vi "Springboard MAIN - App.vi"() -> ()   [LabVIEW 2022 SP3, in "Springboard TLB`.lvlib" / "Springboard TLB`.lvclass"]
uses:
  Springboard TLB`.lvclass
  Application Components/Trigger API/System Trigger.ctl
  State Machine/State.ctl
  Core Components/Error Handler/TLB` Error Handler.lvclass
  Application Components/Configuration/Springboard Station Configuration.lvclass
  Springboard TLB`.lvclass/Springboard TLB`.ctl
  <vilib>/Utility/sysdir.llb/System Directory Type.ctl
  <vilib>/Utility/error.llb/Trim Whitespace One-Sided.vi
  <vilib>/Utility/error.llb/Error Cluster From Error Code.vi
  <vilib>/ErrorRing/Error Ring.xnode
  <vilib>/regexp/Match Regular Expression.xnode
  Application Components/Trigger API/Springboard Trigger API.lvlib
  Springboard TLB`.lvlib
  Core Components/Actions/Actions.lvlib
  Core Components/Dependencies/TLB`_Dependencies.lvlib
  <vilib>/Utility/config.llb/NI_LVConfig.lvlib
panel:
  out "Application Name":string
  out "Application:All Libraries in Application Instance":string[](array[string])
  in  "Library Path":path=path "C:/Program Files (x86)/National Instruments/LabVIEW 2018/project/TLB`/_Dependencies/TLB` Template"
  in  "Add to Project":u16(ring)=2 items=["TLB` Springboard.lvproj", "Untitled Project 14", "< Create In New Project... >"]
  in  "Cancel":bool
  in  "Build":bool
  in  "New TLB Name":string
  in  "Destination Folder":path=path "C:/Users/Public/Documents"
  out "error out":errorcluster
  out "State":string
  out "Status":string
  # "Description"
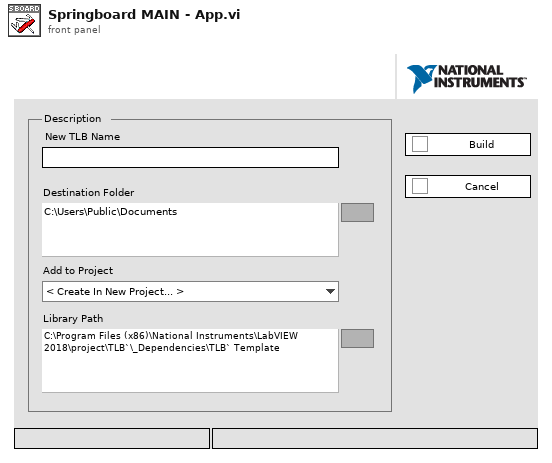
[diagram p1: front panel]
types:
  T1 = typedef "Springboard TLB`.lvlib/Springboard TLB`.lvclass/State.ctl" = enum16{"<Startup>", "Idle", "Evaluate Build Directory", "Creating", "Evaluate Build", "<Shutdown>", "<Error>"}
  T2 = enum16{"Close Display", "Clear References", "Close Error Handler"}
  T3 = enum16{"Clear SR", "Set Display", "Set Shifter", "Initialize Events", "Init Q"}
  T4 = typedef "Springboard TLB`.lvlib/Springboard Trigger API.lvlib/System Trigger.ctl" = enum16{"<None>", "<Return to Safe State Actions>", "<Cache User Parameters>", "<Close Application>", "<Error>", "Create New", "Abort Creation", "Cancel"}
  T5 = typedef "Springboard TLB`.lvlib/_UI CORE Event References.ctl" = cluster{"Exit Event":refnum<user-event>, "State Indicator":refnum<user-event>, "Status Indicator":refnum<user-event>}
  T6 = typedef "Springboard TLB`.lvlib/_UI APP Event References.ctl" = cluster{"Exit Event":refnum<user-event>, "Application Name":refnum<user-event>}
  T7 = enum8{"Enabled", "Disabled", "Disabled and Grayed Out"}
  T8 = typedef "System Directory Type.ctl" = i32
  T9 = typedef "NI_LVConfig.lvlib/Config Data RefNum.ctl" = refnum<k1>
  T10 = enum32{"Invalid", "Standard", "Closed", "Hidden", "Minimized", "Maximized"}
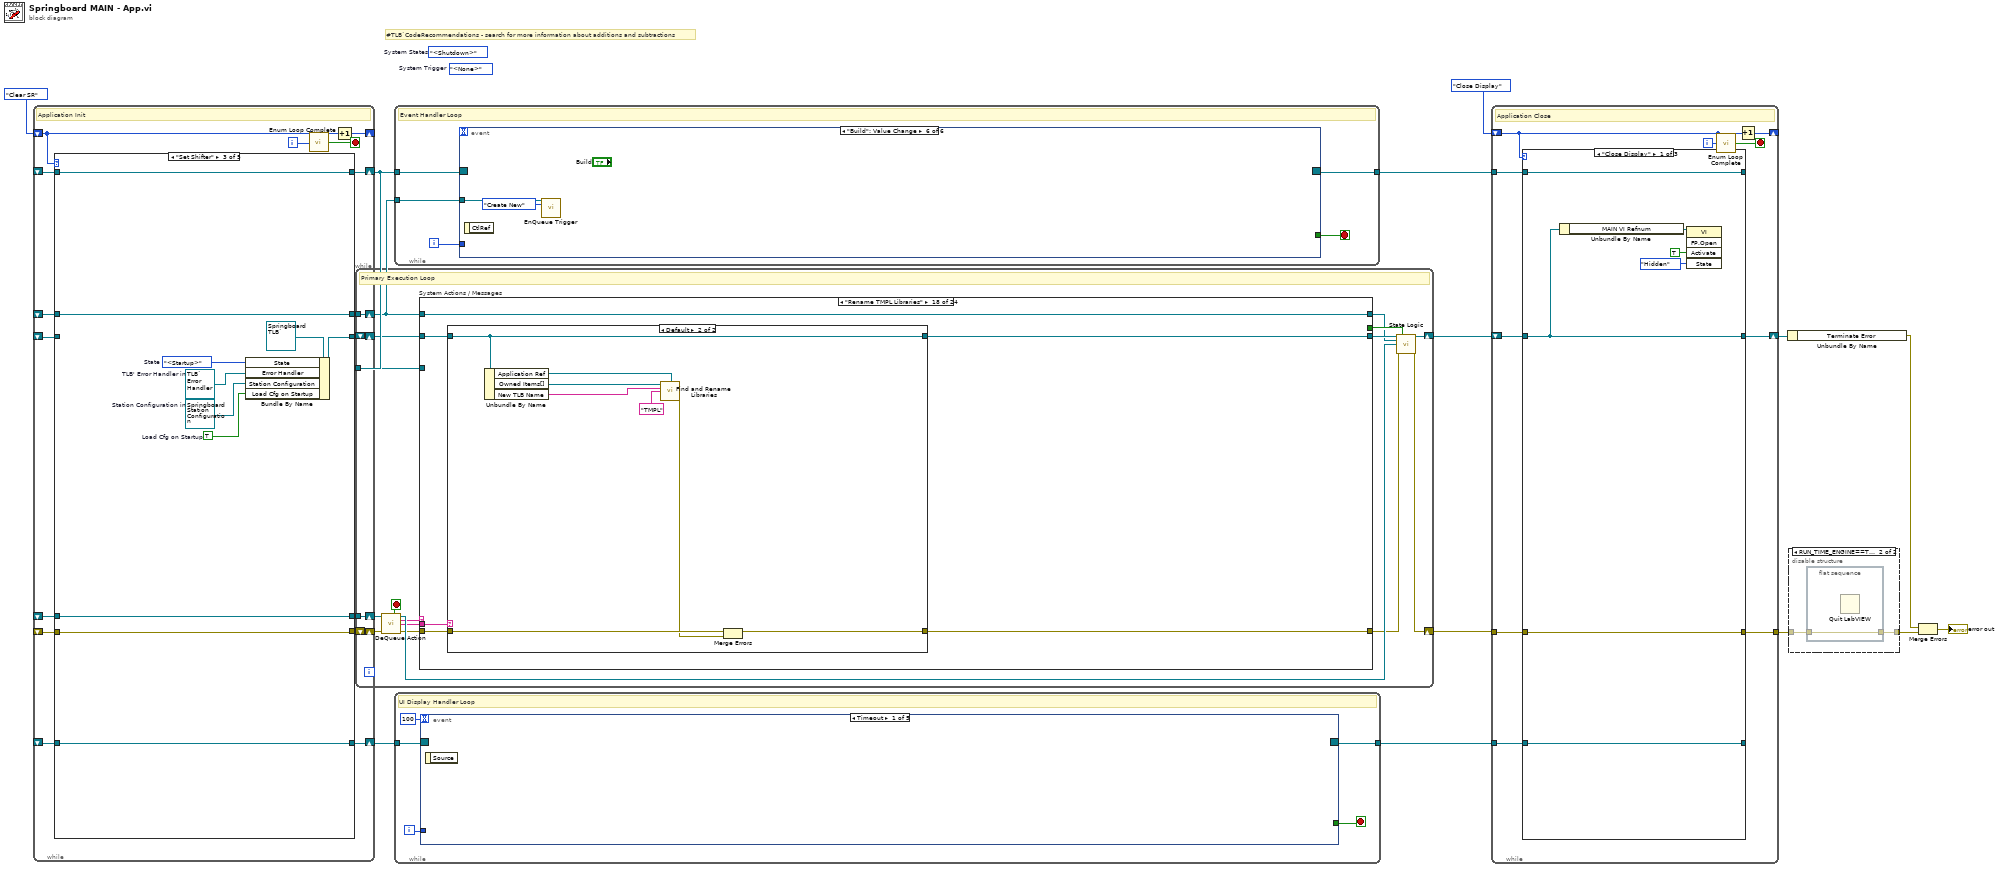
[diagram p0: block diagram]
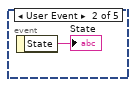
[diagram p2: hidden frame]
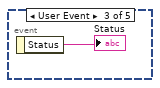
[diagram p3: hidden frame]
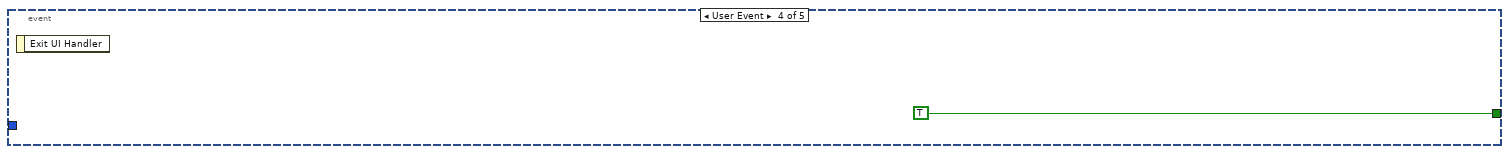
[diagram p4: hidden frame]
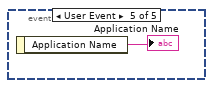
[diagram p5: hidden frame]
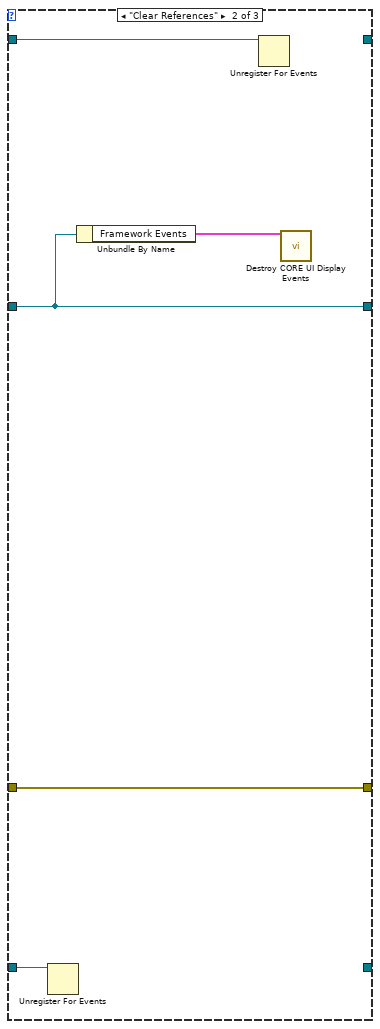
[diagram p7: hidden frame]
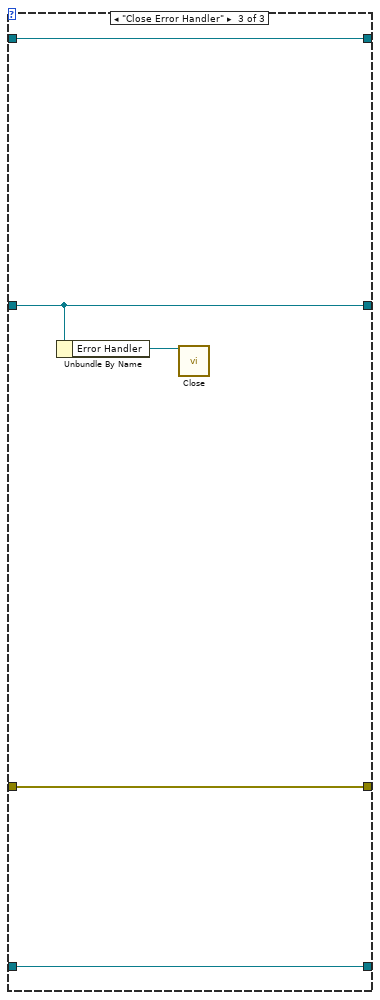
[diagram p8: hidden frame]
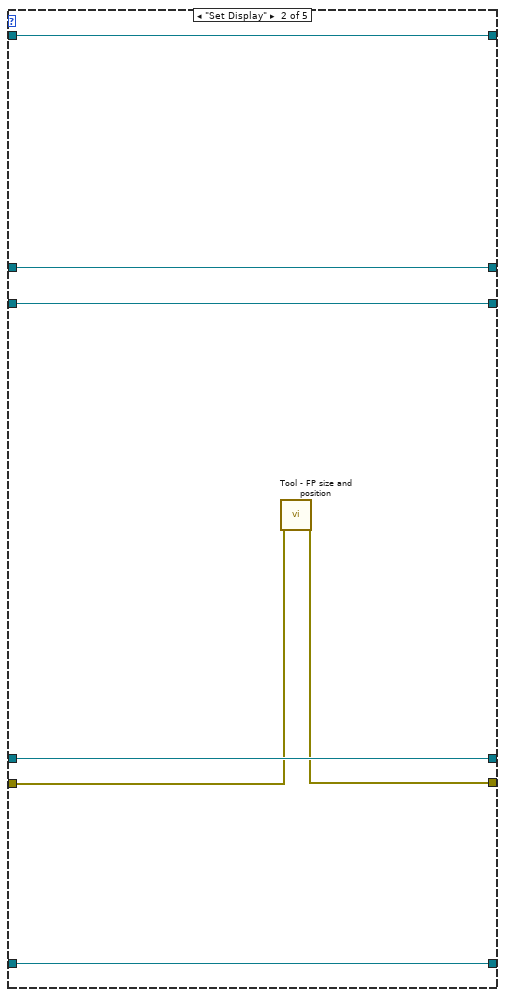
[diagram p10: hidden frame]
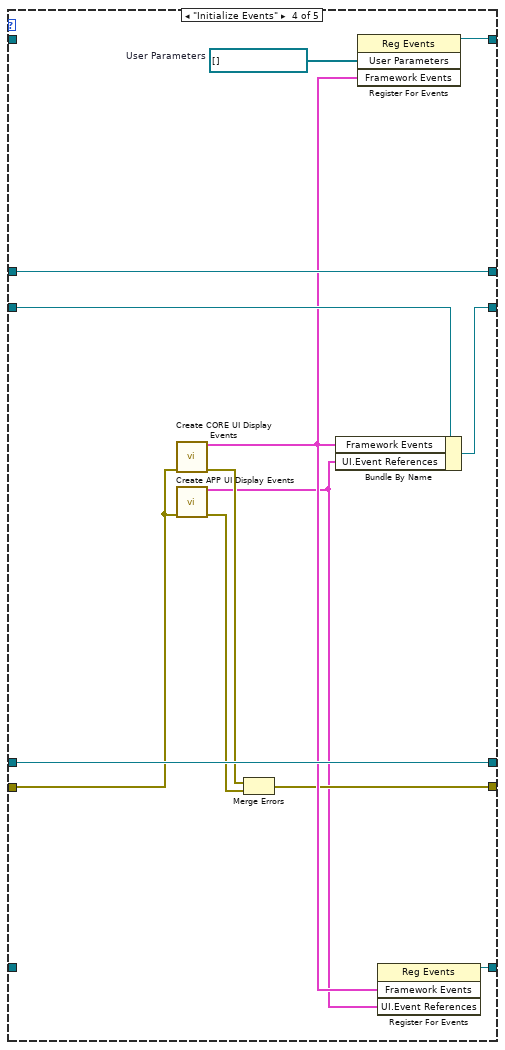
[diagram p11: hidden frame]
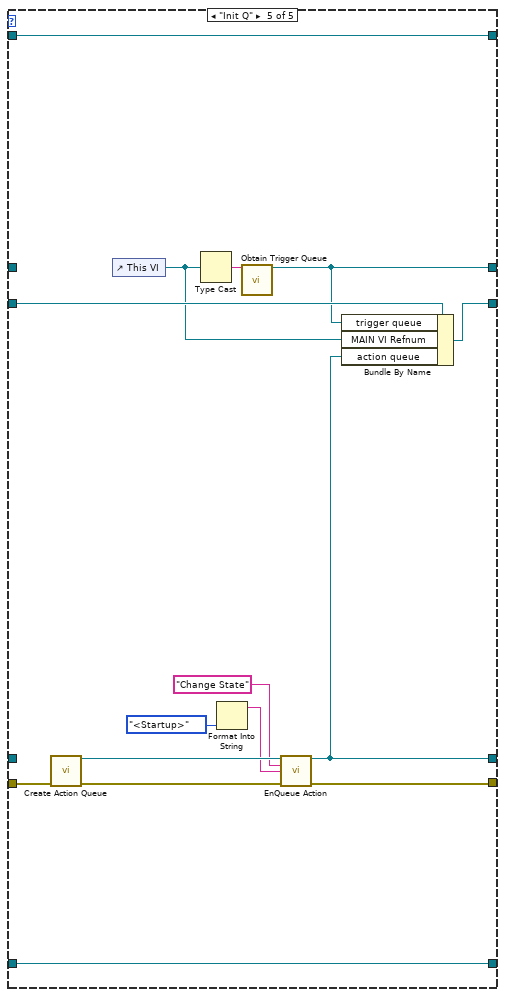
[diagram p12: hidden frame]
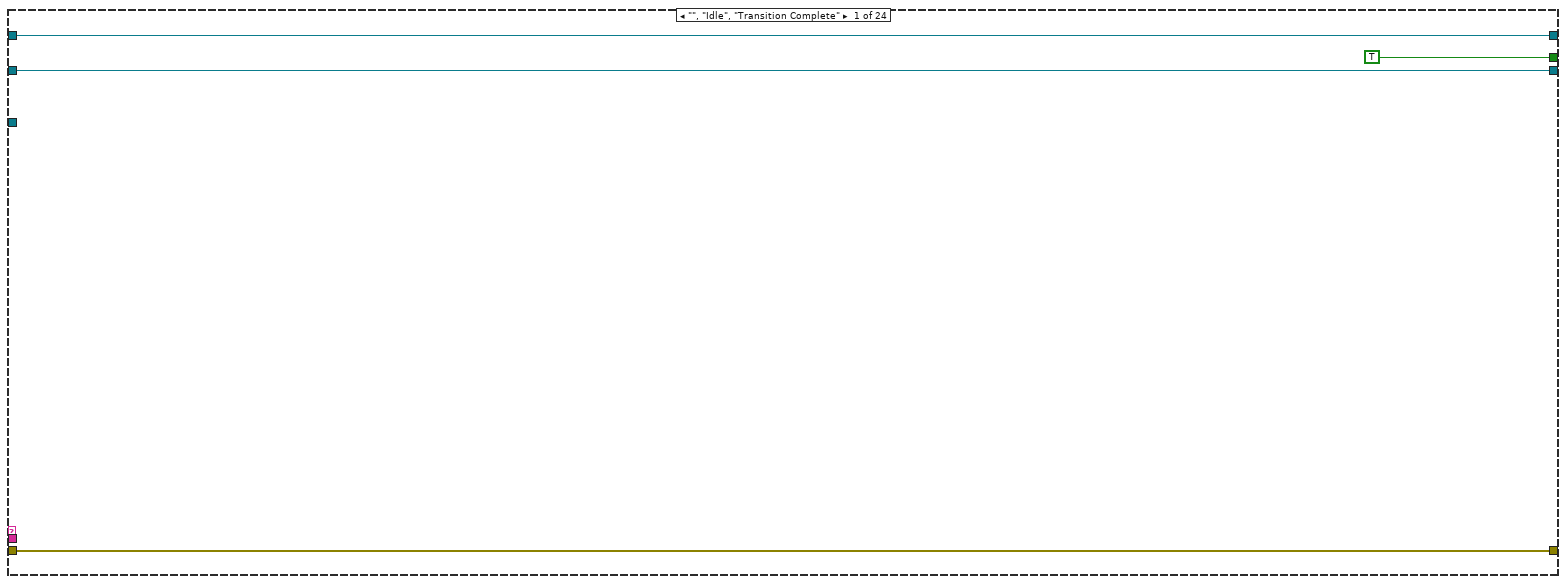
[diagram p13: hidden frame]
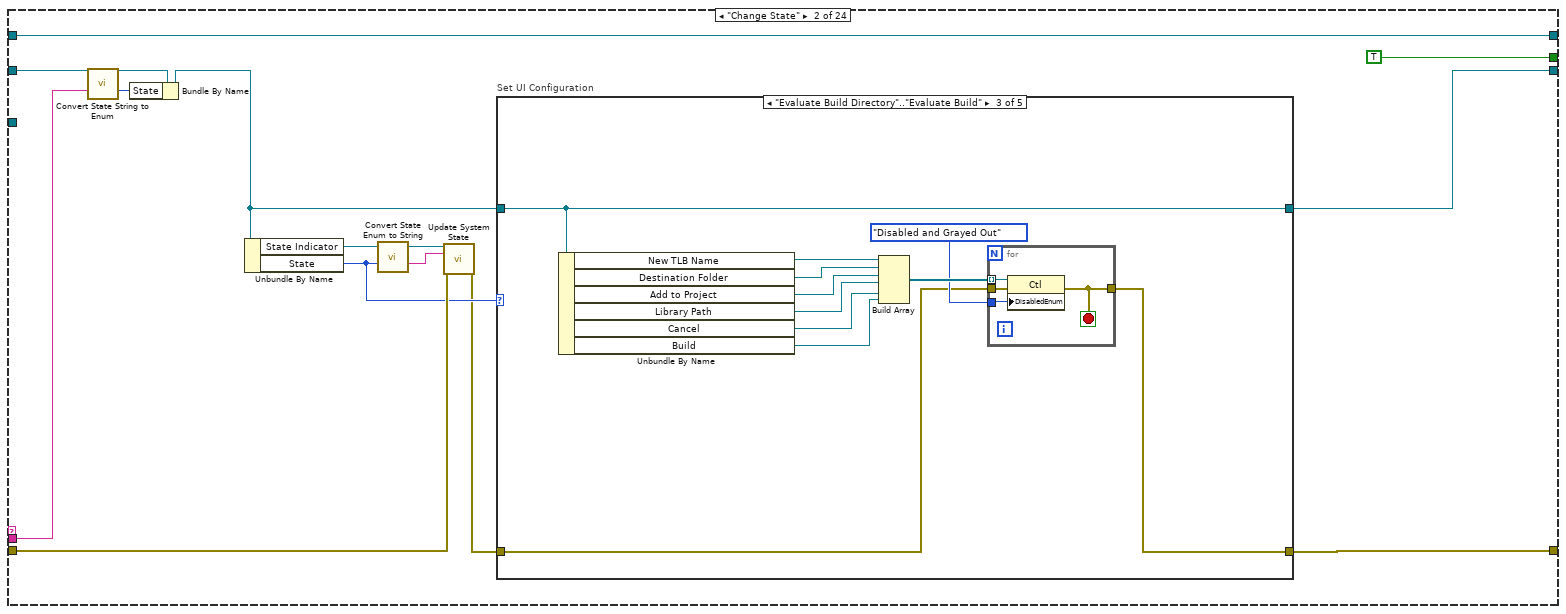
[diagram p14: hidden frame]
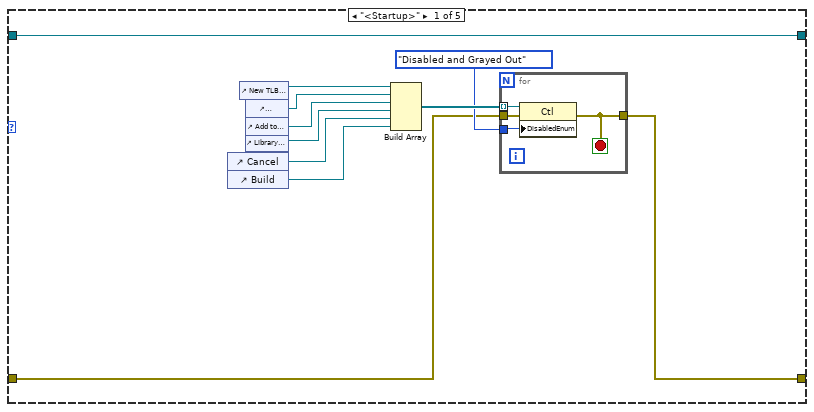
[diagram p15: hidden frame]
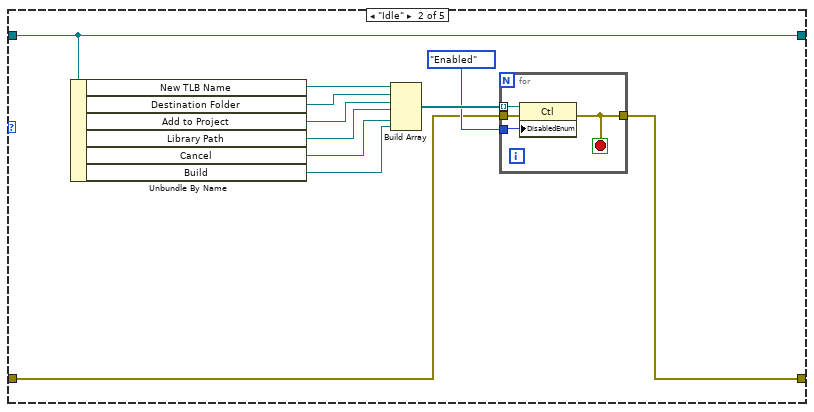
[diagram p16: hidden frame]
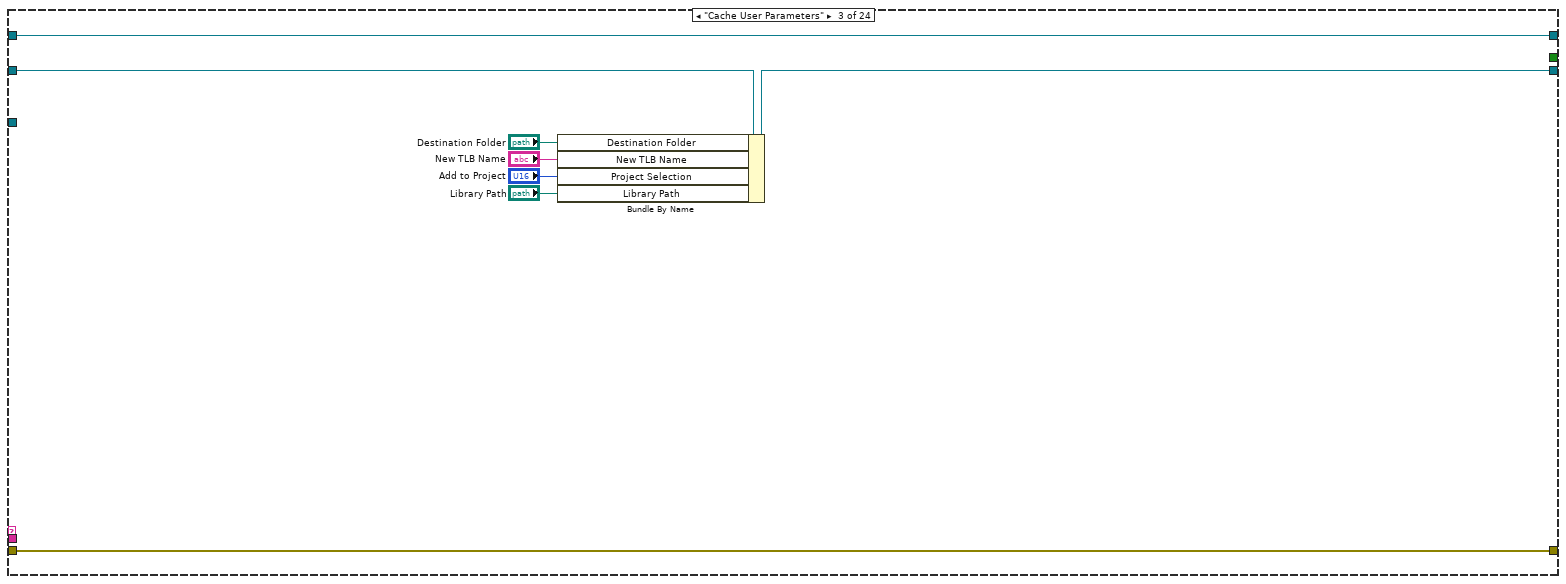
[diagram p19: hidden frame]
diagram:
  (unwired) State."<Shutdown>"  # System States
  (unwired) System_Trigger."<None>"  # System Trigger
  # "#TLB`CodeRecommendations - search for more information about additions and subtractions"
  n1 = while {
    shift-right: [w29] -> _
    shift-left: T3."Clear SR" -> [w18]
    shift-right: [w33] -> w17
    shift-left: _ -> [w28]
    shift-right: [w30] -> w12
    shift-left: _ -> [w27]
    shift-right: [w32] -> w11
    shift-left: _ -> [w26]
    shift-right: [w31] -> w10
    shift-left: _ -> [w25]
    shift-right: [w24] -> w6
    shift-left: _ -> [w23]
    shift-right: [w22] -> w9
    shift-left: _ -> [w21]
    i -> [w19]
    stop <- w20 stop-if-true
    # "Application Init"
    n2 = case shown="\"Set Shifter\"" w18 {
      tunnel: [_ w38 w51 w64 w68] -> w33
      tunnel: [_ w36 w50 w54 w72] -> w30
      tunnel: [_ w40 w46 w62 w77] -> w31
      tunnel: [_ w39 w49 w61 w79] -> w32
      tunnel: w28 -> [_ w38 w51 w64 _]
      tunnel: w27 -> [_ w37 w50 w53 w74]
      tunnel: w26 -> [_ w39 w49 _ w79]
      tunnel: w25 -> [_ w40 _ w63 w78]
      tunnel: [_ w35 w48 w60 w69] -> w24
      tunnel: w23 -> [_ w35 w48 w60 _]
      tunnel: [_ w34 w44 w58 w75] -> w22
      tunnel: w21 -> [_ w34 w44 _ w75]
      frame "Clear SR" {
      }
      frame "Set Display" {
        n3 = call "Tool - FP size and position.vi"("error in (no error)"=w37) -> ("error out"=w36:errorcluster)  [unwired: 17 in, 1 out]
      }
      frame "Set Shifter" {
        w41 = TRUE  # Load Cfg on Startup
        w42 = refnum<class "Springboard Station Configuration.lvclass"> refnum  # Station Configuration in
        w43 = refnum<class "TLB` Error Handler.lvclass"> refnum  # TLB' Error Handler in
        w47 = State."<Startup>"  # State
        n4 = Bundle By Name(cluster=refnum<class "Springboard TLB`.lvclass"> refnum ("TLB` Template.lvlib:TLB' Template.lvclass"), "State"=w47, "Error Handler"=w43, "Station Configuration"=w42, "Load Cfg on Startup"=w41) -> (w46:refnum<class "Springboard TLB`.lvclass">)
      }
      frame "Initialize Events" {
        w59 = refnum<vi>[] []  # User Parameters
        n5 = call "Create CORE UI Display Events.vi"("error in"=w53) -> ("Framework Events"=w57:T5, "error out"=w56:errorcluster)  [unwired: 13 in]
        n6 = call "Create APP UI Display Events.vi"("error in"=w53) -> ("UI.Event References"=w52:T6, "error out"=w55:errorcluster)  [unwired: 13 in]
        n7 = Merge Errors(w56, w55) -> (w54:errorcluster)
        n8 = Bundle By Name(cluster=w63, "Framework Events"=w57, "UI.Event References"=w52) -> (w62:refnum<class "Springboard TLB`.lvclass">)
        n9 = register-events(w59, w57) -> (reference out=w61:refnum<event-registration>)  [unwired: 2 in, 1 out]
        n10 = register-events(w57, w52) -> (reference out=w58:refnum<event-registration>)  [unwired: 2 in, 1 out]
      }
      frame "Init Q" {
        n11 = call "Create Action Queue.vi"("error in"=w74) -> ("action queue out"=w71:refnum<queue>, "error out"=w73:errorcluster)  [unwired: 13 in]
        n12 = control-ref of="This VI"() -> (w76:refnum<vi>)
        n13 = Type Cast(x=w76) -> (*(type *) &x=w70:string)  [unwired: 1 in]
        n14 = Format Into String(State."<Startup>" ("State")) -> (resulting string=w65:string)  [unwired: 3 in, 1 out]
        n15 = call "Obtain Trigger Queue.vi"("trigger queue name"=w70) -> ("trigger queue out"=w69:refnum<queue>)  [unwired: 13 in, 1 out]
        n16 = call "EnQueue Action.vi"("action queue in"=w71, "action"="Change State" ("Message Name"), "data in"=w65, "error in"=w73) -> ("action queue out"=w68:refnum<queue>, "error out"=w72:errorcluster)  [unwired: 10 in]
        n17 = Bundle By Name(cluster=w78, "trigger queue"=w69, "MAIN VI Refnum"=w76, "action queue"=w68) -> (w77:refnum<class "Springboard TLB`.lvclass">)
      }
    }
    n18 = call "Enum Loop Complete.vi"("Current State Enum"=w18, "Itteration"=w19) -> ("Loop Complete?"=w20:bool)  [unwired: 12 in, 1 out]
    n19 = Increment(x=w18) -> (x+1=w29:T3)
  }
  n20 = while {
    shift-right: [w90] -> w8
    shift-left: w12 -> [w85]
    shift-right: [w92] -> w13
    shift-left: w10 -> [w94]
    tunnel: w17 -> [w86]
    tunnel: w11 -> [w93]
    tunnel: w6 -> [w89]
    stop <- w84 stop-if-true
    # "Primary Execution Loop"
    n21 = call "DeQueue Action.vi"("action queue in"=w86, "error in"=w85) -> ("exit?"=w84:bool, "action queue out"=w95:refnum<queue>, "action"=w82:string, "action value"=w80:string, "error out"=w83:errorcluster)  [unwired: 8 in, 1 out]
    n22 = case "System Actions / Messages" shown="\"Rename TMPL Libraries\"" w82 {
      selector: w82 -> [_ _ _ _ _ _ _ _ _ _ _ _ _ _ _ _ _ _ _ _ _ _ _ w720]
      tunnel: [w99 w110 w168 w172 w173 w182 w197 w207 w231 w263 w269 w271 w389 w419 w592 w638 w661 w674 w692 w697 w702 w703 w715 w719] -> w87
      tunnel: w83 -> [w99 w109 w168 w172 w173 w185 w197 w212 w234 w261 w269 w274 w390 w420 w595 w637 w662 w677 w692 w696 w702 w704 w716 _]
      tunnel: w94 -> [w96 w108 w166 w171 w176 w183 w199 w215 w235 w257 w268 w273 w392 w422 w594 w640 w663 w678 w691 w699 w701 w707 w718 w722]
      tunnel: [w96 w104 w169 w171 w175 w188 w202 w214 w225 w258 w268 w272 w391 w421 w593 w639 w659 w675 w691 w699 w701 w706 w717 w722] -> w91
      tunnel: w93 -> [_ _ _ _ _ _ w200 _ _ _ _ _ _ _ _ _ _ _ _ _ _ _ _ _]
      tunnel: [w97 w111 w167 w170 w177 w189 w201 w220 w239 w266 w267 w270 w393 w423 w596 w641 w664 w679 w690 w694 w700 w710 w711 w721] -> w81
      tunnel: w89 -> [w97 w111 w167 w170 w177 w189 w201 w220 w239 w266 w267 w270 w393 w423 w596 w641 w664 w679 w690 w694 w700 w710 w711 w721]
      tunnel: [TRUE TRUE _ _ _ _ _ _ _ _ _ _ _ _ _ _ _ _ _ _ _ _ _ _] -> w88
      tunnel: w80 -> [_ w107 _ _ _ _ _ _ _ _ _ w275 w388 w418 w591 w636 w660 w676 _ _ _ _ _ _]
      frame "", "Idle", "Transition Complete" {
      }
      frame "Change State" {
        n23 = call "Convert State String to Enum.vi"("state in"=w107) -> ("state out"=w106:T1)  [unwired: 13 in, 1 out]
        n24 = Bundle By Name(cluster=w108, "State"=w106) -> (w105:refnum<class "Springboard TLB`.lvclass">)
        n25 = Unbundle By Name(w105) -> ("State Indicator"=w100:refnum<user-event>, "State"=w103:T1)
        n26 = call "Convert State Enum to String.vi"("state in"=w103) -> ("state out"=w101:string)  [unwired: 13 in, 1 out]
        n27 = call "Update System State.vi"("State Indicator"=w100, "system state message"=w101, "error in"=w109) -> ("error out"=w102:errorcluster)  [unwired: 12 in]
        n28 = case "Set UI Configuration" shown="\"Evaluate Build Directory\"..\"Evaluate Build\"" w103 {
          tunnel: [w120 w129 w144 w158 w161] -> w110
          tunnel: w102 -> [w119 w128 w143 w158 w161]
          tunnel: [w123 w138 w153 w159 w160] -> w104
          tunnel: w105 -> [w123 w138 w153 w159 w160]
          frame "<Startup>" {
            n29 = control-ref of="Cancel"() -> (w114:refnum<vi>)
            n30 = control-ref of="Build"() -> (w113:refnum<vi>)
            n31 = control-ref of="New TLB Name"() -> (w118:refnum<vi>)
            n32 = control-ref of="Destination Folder"() -> (w117:refnum<vi>)
            n33 = control-ref of="Add to Project"() -> (w116:refnum<vi>)
            n34 = control-ref of="Library Path"() -> (w115:refnum<vi>)
            n35 = Build Array(w118, w117, w116, w115, w114, w113) -> (w122:refnum<vi>[])
            n36 = for {
              tunnel: w122 -> [w127] mode=indexing
              tunnel: T7."Disabled and Grayed Out" ("Disabled") -> [w126]
              tunnel: w119 -> [w125]
              tunnel: [w124] -> w120
              stop <- w124 stop-if-true
              n37 = property class="Ctl"(reference=w127, error in=w125, "DisabledEnum"=w126) -> (error out=w124:errorcluster)  [unwired: 1 out]
            }
          }
          frame "Idle" {
            n38 = Unbundle By Name(w138) -> ("New TLB Name"=w137:refnum<vi>, "Destination Folder"=w136:refnum<vi>, "Add to Project"=w135:refnum<vi>, "Library Path"=w134:refnum<vi>, "Cancel"=w133:refnum<vi>, "Build"=w132:refnum<vi>)
            n39 = Build Array(w137, w136, w135, w134, w133, w132) -> (w131:refnum<vi>[])
            n40 = for {
              tunnel: w131 -> [w142] mode=indexing
              tunnel: T7."Enabled" ("Disabled") -> [w141]
              tunnel: w128 -> [w140]
              tunnel: [w139] -> w129
              stop <- w139 stop-if-true
              n41 = property class="Ctl"(reference=w142, error in=w140, "DisabledEnum"=w141) -> (error out=w139:errorcluster)  [unwired: 1 out]
            }
          }
          frame "Evaluate Build Directory".."Evaluate Build" {
            n42 = Unbundle By Name(w153) -> ("New TLB Name"=w152:refnum<vi>, "Destination Folder"=w151:refnum<vi>, "Add to Project"=w150:refnum<vi>, "Library Path"=w149:refnum<vi>, "Cancel"=w148:refnum<vi>, "Build"=w147:refnum<vi>)
            n43 = Build Array(w152, w151, w150, w149, w148, w147) -> (w146:refnum<vi>[])
            n44 = for {
              tunnel: w146 -> [w157] mode=indexing
              tunnel: T7."Disabled and Grayed Out" ("Disabled") -> [w156]
              tunnel: w143 -> [w155]
              tunnel: [w154] -> w144
              stop <- w154 stop-if-true
              n45 = property class="Ctl"(reference=w157, error in=w155, "DisabledEnum"=w156) -> (error out=w154:errorcluster)  [unwired: 1 out]
            }
          }
          frame "<Error>" {
          }
          frame "<Shutdown>" {
          }
        }
      }
      frame "Cache User Parameters" {
        n46 = Bundle By Name(cluster=w166, "Destination Folder"="Destination Folder", "New TLB Name"="New TLB Name", "Project Selection"="Add to Project", "Library Path"="Library Path") -> (w169:refnum<class "Springboard TLB`.lvclass">)
      }
      frame "/*********INITialize********/" {
      }
      frame "INIT::Load Application Base Path" {
        n47 = disable-structure shown="Default" {
          disable-tunnel: [w178 w180] -> w174
          frame condition #0 (active) {
            n48 = Current VI's Path() -> (path=w179:path)
            n49 = Strip Path(path=w179) -> (stripped path=w178:path)  [unwired: 1 out]
          }
          frame condition #1 {
            n50 = call <vilib>:"Application Directory.vi"() -> ("Application Directory"=w180:path)
          }
        }
        n51 = Bundle By Name(cluster=w176, "Application Base Path"=w174) -> (w175:refnum<class "Springboard TLB`.lvclass">)
      }
      frame "INIT::Initialize Error Handler" {
        n52 = Unbundle By Name(w183) -> ("Application Base Path"=w190:path)
        n53 = Unbundle By Name(w183) -> ("Error Handler"=w184:refnum<class "TLB` Error Handler.lvclass">)
        n54 = Build Path(base path=w190, name or relative path="System Level Errors\\System Errors.txt") -> (appended path=w186:path)
        n55 = call-dynamic "Open.vi"("error handler in"=w184, "error log path in"=w186, "error in"=w185) -> ("error handler out"=w187:refnum<class "TLB` Error Handler.lvclass">, "error out"=w182:errorcluster)  [unwired: 11 in]
        n56 = Bundle By Name(cluster=w183, "Error Handler"=w187) -> (w188:refnum<class "Springboard TLB`.lvclass">)
      }
      frame "INIT::Register User Parameters" {
        n57 = control-ref of="Cancel"() -> (w192:refnum<vi>)
        n58 = control-ref of="Build"() -> (w191:refnum<vi>)
        n59 = control-ref of="New TLB Name"() -> (w196:refnum<vi>)
        n60 = control-ref of="Destination Folder"() -> (w195:refnum<vi>)
        n61 = control-ref of="Add to Project"() -> (w194:refnum<vi>)
        n62 = control-ref of="Library Path"() -> (w193:refnum<vi>)
        n63 = Build Array(w196, w195, w194, w193) -> (w198:refnum<vi>[])
        n64 = register-events(reference=w200, w198) -> ()  [unwired: 2 in, 2 out]
        n65 = Bundle By Name(cluster=w199, "User Parameter Controls"=w198, "New TLB Name"=w196, "Destination Folder"=w195, "Add to Project"=w194, "Library Path"=w193, "Cancel"=w192, "Build"=w191) -> (w202:refnum<class "Springboard TLB`.lvclass">)
      }
      frame "INIT::Project Ring Initialize" {
        n66 = property class="App"(error in=w212) -> (error out=w211:errorcluster, "App.AllMyLibses"=→"Application:All Libraries in Application Instance":string[])  [unwired: 1 in, 1 out]
        n67 = property class="App"(error in=w211) -> (error out=w210:errorcluster, "Project"=w217:refnum<vi>[])  [unwired: 1 in, 1 out]
        n68 = Bundle By Name(cluster=w215, "Projects In Memory"=w217) -> (w214:refnum<class "Springboard TLB`.lvclass">)
        n69 = for {
          tunnel: w217 -> [w224] mode=indexing
          tunnel: [w223] -> w219 mode=indexing
          tunnel: w210 -> [w222]
          tunnel: [w221] -> w209 mode=indexing
          n70 = property class="Project"(reference=w224, error in=w222) -> (error out=w221:errorcluster, "Name"=w223:string)  [unwired: 1 out]
        }
        n71 = Unbundle By Name(w214) -> ("Add to Project"=w213:refnum<vi>)
        n72 = Merge Errors(w209) -> (w208:errorcluster)
        n73 = Build Array (concatenate)(w219, "< Create In New Project... >") -> (w206:string[])
        n74 = Array Size(array=w206) -> (size(s)=w205:i32)
        n75 = Decrement(x=w205) -> (x-1=w204:i32)
        n76 = To Unsigned Word Integer(number=w204) -> (unsigned 16bit integer=w203:u16)
        n77 = property class="Ring (strict)"(reference=w213, error in=w208, "Strings []"=w206, "Value"=w203) -> (error out=w207:errorcluster)  [unwired: 1 out]
      }
      frame "INIT::FP Values" {
        w229 = T8 2 items=["User Home"=0, "User Desktop"=1, "User Documents"=2, "User Application Data"=3, "User Preferences"=4, "User Temporary"=5, "Public Documents"=6, "Public Application Data"=7, "Public Preferences"=8, "Public Cache"=13, "System Core Libraries"=9, "System Installed Libraries"=10, "Application Files"=11, "Boot Volume Root"=12] ("system directory type")
        # "empty original TLB` template name"
        # "#TLB`CodeRecommendations - initialize FP values here"
        n78 = Unbundle By Name(w235) -> ("Library Path"=w238:refnum<vi>, "New TLB Name"=w237:refnum<vi>)
        n79 = Build Array(w238) -> (w232:refnum<vi>[])
        n80 = property class="Str"(reference=w237, error in=w234, "Value"="") -> (error out=w233:errorcluster)  [unwired: 1 out]
        n81 = in-place {
          in-place-border: w233 -> [w246]
          in-place-border: w232 -> [w249]
          in-place-border: [w241] -> w228
          n82 = in-place-cluster #1(w235) -> ("Application Name"=w245:refnum<user-event>, "Station Configuration"=w256:refnum<class "Springboard Station Configuration.lvclass">)
          n83 = call-dynamic "Get Application Name.vi"("error in"=w246, "Springboard Station Configuration in"=w256) -> ("error out"=w255:errorcluster, "Application Name"=w243:string, "Springboard Station Configuration out"=w254:refnum<class "Springboard Station Configuration.lvclass">)  [unwired: 7 in]
          n84 = call-dynamic "Get Cache User Parameters File Path.vi"("error in (no error)"=w255, "Springboard Station Configuration in"=w254) -> ("error out"=w252:errorcluster, "station config INI path"=w253:path, "Springboard Station Configuration out"=w240:refnum<class "Springboard Station Configuration.lvclass">)  [unwired: 7 in]
          n85 = call <vilib>:"Open Config Data.vi"("error in (no error)"=w252, "configuration file path"=w253) -> ("error out"=w251:errorcluster, "refnum"=w250:T9)  [unwired: 7 in, 1 out]
          n86 = call "Read Anything.vi"("refnum"=w250, "user parameter references in"=w249, "error in"=w251) -> ("refnum out"=w247:T9, "error out"=w248:errorcluster)  [unwired: 11 in]
          n87 = call <vilib>:"Close Config Data.vi"("error in (no error)"=w248, "refnum"=w247) -> ("error out"=w242:errorcluster)  [unwired: 8 in, 1 out]
          n88 = Generate User Event(user event=w245, event data cluster=w243, error in=w242) -> (user event out=w244:refnum<user-event>, error out=w241:errorcluster)  [unwired: 1 in]
          n89 = in-place-cluster #1("Application Name"=w244, "Station Configuration"=w240) -> (w227:refnum<class "Springboard TLB`.lvclass">)
        }
        n90 = Unbundle By Name(w227) -> ("Destination Folder"=w230:refnum<vi>)
        n91 = call <vilib>:"Get System Directory.vi"("system directory type"=w229) -> ("system directory"=w226:path)  [unwired: 10 in]
        n92 = Bundle By Name(cluster=w227, "User Directory"=w226) -> (w225:refnum<class "Springboard TLB`.lvclass">)
        n93 = property class="Path"(reference=w230, error in=w228, "Value"=w226) -> (error out=w231:errorcluster)  [unwired: 1 out]
      }
      frame "CFG::Load Station Configuration" {
        n94 = Unbundle By Name(w257) -> ("Application Base Path"=w265:path)
        n95 = Unbundle By Name(w257) -> ("Station Configuration"=w260:refnum<class "Springboard Station Configuration.lvclass">)
        n96 = Build Path(base path=w265, name or relative path="System Configuration\\Station Configuration.ini") -> (appended path=w262:path)
        n97 = call-dynamic "Load Configuration.vi"("INI Station Configuration in"=w260, "INI file path in"=w262, "error in"=w261) -> ("INI Station Configuration out"=w259:refnum<class "Springboard Station Configuration.lvclass">, "error out"=w263:errorcluster)  [unwired: 11 in]
        n98 = Bundle By Name(cluster=w257, "Station Configuration"=w259) -> (w258:refnum<class "Springboard TLB`.lvclass">)
      }
      frame "/*********PRImary EXEcution********/" {
      }
      frame "Validate Destination Directory" {
        n99 = case shown="Default" w275 {
          tunnel: w274 -> [w281 w294]
          tunnel: w273 -> [w285 w293]
          tunnel: [w276 w299] -> w271
          tunnel: [w285 w292] -> w272
          tunnel: w270 -> [_ w300]
          frame "Undo" {
            n100 = Unbundle By Name(w285) -> ("Destination Folder"=w284:refnum<vi>, "User Directory"=w283:path, "Destination Folder"=w282:path)
            n101 = call <vilib>:"Check if File or Folder Exists.vi"("error in (no error)"=w281, "path"=w282) -> ("error out"=w278:errorcluster, "file or folder exists?"=w280:bool, "dup path"=w279:path)  [unwired: 7 in]
            n102 = case shown="True" w280 {
              tunnel: w279 -> [_ w290]
              tunnel: w278 -> [w286 w289]
              tunnel: [w286 w288] -> w277
              frame False {
              }
              frame True {
                n103 = Delete(path (use dialog)=w290, entire hierarchy (F)=TRUE, error in=w289) -> (error out=w288:errorcluster)  [unwired: 2 in, 2 out]
              }
            }
            n104 = property class="Path"(reference=w284, error in=w277, "Value"=w283) -> (error out=w276:errorcluster)  [unwired: 1 out]
          }
          frame Default {
            # "an empty TLB` Name isn't valid"
            n105 = Unbundle By Name(w293) -> ("Library Path"=w301:path, "Destination Folder"=w298:path, "New TLB Name"=w295:string, "User Directory"=w291:path)
            n106 = Equal?(x=w295, y="") -> (x = y?=w296:bool)
            n107 = case shown="False" w296 {
              tunnel: w301 -> [w320 _]
              tunnel: w300 -> [w316 w380]
              tunnel: [w315 w376] -> w299
              tunnel: w298 -> [w305 _]
              tunnel: w295 -> [w313 _]
              tunnel: w294 -> [w310 w379]
              tunnel: w293 -> [w304 w382]
              tunnel: [w303 w382] -> w292
              tunnel: w291 -> [w302 _]
              frame False {
                # "if the new installation directory is empty go ahead\nand attempt to create the new TLB` Template"
                # "assist user in putting files into a specific directory \nopposed to default User Documents append new \nTLB` name to User Documents Path"
                n108 = Equal?(x=w305, y=w302) -> (x = y?=w312:bool)
                n109 = case shown="True" w312 {
                  tunnel: w305 -> [w356 w365]
                  tunnel: [w356 w357] -> w314
                  tunnel: w313 -> [_ w364]
                  tunnel: [w355 w362] -> w311
                  tunnel: w310 -> [w355 w360]
                  frame False {
                  }
                  frame True {
                    n110 = Build Path(base path=w365, name or relative path=w364) -> (appended path=w363:path)
                    n111 = call <vilib>:"Check if File or Folder Exists.vi"("error in (no error)"=w360, "path"=w363) -> ("error out"=w358:errorcluster, "file or folder exists?"=w359:bool, "dup path"=w361:path)  [unwired: 7 in]
                    n112 = case shown="True" w359 {
                      tunnel: [w369 w371] -> w357
                      tunnel: [w368 w370] -> w362
                      tunnel: w361 -> [w367 w371]
                      tunnel: w358 -> [w366 w370]
                      frame False {
                        n113 = Create Folder(path (use dialog)=w367, error in=w366) -> (created path=w369:path, error out=w368:errorcluster)  [unwired: 1 in, 1 out]
                      }
                      frame True {
                      }
                    }
                  }
                }
                n114 = Strip Path(path=w320) -> (stripped path=w309:path)  [unwired: 1 out]
                n115 = List Folder(path=w314, error in=w311) -> (folder names=w307:string[], error out=w319:errorcluster)  [unwired: 2 in, 2 out]
                n116 = List Folder(path=w309, error in=w319) -> (filenames=w308:string[], error out=w317:errorcluster)  [unwired: 2 in, 2 out]
                n117 = Empty Array?(array=w307) -> (empty?=w306:bool)
                n118 = for {
                  tunnel: w307 -> [w372] mode=indexing
                  shift-right: [w375] -> _
                  shift-left: w308 -> [w375]
                  tunnel: [w372] -> w318
                  stop <- w373 stop-if-true
                  n119 = Search 1D Array(1D array=w375, element=w372) -> (index of element=w374:i32)  [unwired: 1 in]
                  n120 = Greater Or Equal To 0?(x=w374) -> (x >= 0?=w373:bool)
                }
                n121 = case shown="False" w306 {
                  tunnel: w318 -> [w333 _]
                  tunnel: w317 -> [w326 w349]
                  tunnel: w316 -> [w325 w350]
                  tunnel: [w324 w348] -> w315
                  tunnel: w314 -> [w322 w353]
                  tunnel: w304 -> [w323 w354]
                  tunnel: [w321 w352] -> w303
                  frame False {
                    # "if the directory to be created has\nmatching files, give the user a \nchance to avoid overriding files."
                    n122 = Build Path(base path=w322, name or relative path=w333) -> (appended path=w332:path)
                    n123 = Path To String(path=w332) -> (string=w331:string)
                    n124 = Concatenate Strings("A directory structure of " ("string"), w331, " already exists.  Creating the directory here may result in the overriding existing files.  Do you want to continue?" ("string")) -> (w328:string)
                    n125 = Two Button Dialog(message=w328, 1:"No" ("F button name (\"Cancel\")"), 2:"Yes" ("T button name (\"OK\")")) -> (T button?=w327:bool)
                    n126 = case shown="False" w327 {
                      tunnel: w326 -> [w338 w342]
                      tunnel: w325 -> [w339 w343]
                      tunnel: [w337 w341] -> w324
                      tunnel: w323 -> [w336 w347]
                      tunnel: w322 -> [_ w346]
                      tunnel: [w336 w345] -> w321
                      frame False {
                        n127 = call "EnQueue Trigger.vi"("trigger queue in"=w339, "system trigger"=System_Trigger."Abort Creation" ("System Trigger"), "error in"=w338) -> ("error out"=w337:errorcluster)  [unwired: 11 in, 1 out]
                      }
                      frame True {
                        n128 = Bundle By Name(cluster=w347, "Destination Folder"=w346) -> (w345:refnum<class "Springboard TLB`.lvclass">)
                        n129 = call "EnQueue Trigger.vi"("trigger queue in"=w343, "system trigger"=System_Trigger."Create New" ("System Trigger"), "error in"=w342) -> ("error out"=w341:errorcluster)  [unwired: 11 in, 1 out]
                      }
                    }
                  }
                  frame True {
                    n130 = Bundle By Name(cluster=w354, "Destination Folder"=w353) -> (w352:refnum<class "Springboard TLB`.lvclass">)
                    n131 = call "EnQueue Trigger.vi"("trigger queue in"=w350, "system trigger"=System_Trigger."Create New" ("System Trigger"), "error in"=w349) -> ("error out"=w348:errorcluster)  [unwired: 11 in, 1 out]
                  }
                }
              }
              frame True {
                n132 = xnode "Error Ring"() -> ("error out"=w377:errorcluster)
                n133 = call "EnQueue Trigger.vi"("trigger queue in"=w380, "system trigger"=System_Trigger."Abort Creation" ("System Trigger"), "error in"=w379) -> ("error out"=w378:errorcluster)  [unwired: 11 in, 1 out]
                n134 = Merge Errors(w378, w377) -> (w376:errorcluster)
              }
            }
          }
        }
      }
      frame "Get Project References" {
        n135 = case shown="\"Undo\"" w388 {
          tunnel: w392 -> [w394 w399]
          tunnel: [w394 w398] -> w391
          tunnel: w390 -> [w395 w397]
          tunnel: [w395 w396] -> w389
          frame "Undo" {
          }
          frame Default {
            n136 = Unbundle By Name(w399) -> ("Projects In Memory"=w406:refnum<vi>[], "Project Selection"=w408:u16)
            n137 = To Long Integer(number=w408) -> (32bit integer=w404:i32)
            n138 = Array Size(array=w406) -> (size(s)=w407:i32)
            n139 = Less?(x=w404, y=w407) -> (x < y?=w405:bool)
            n140 = case shown="True" w405 {
              tunnel: w404 -> [_ w417]
              tunnel: w406 -> [_ w416]
              tunnel: [w412 w415] -> w403
              tunnel: [w411 w414] -> w400
              tunnel: w397 -> [w409 w414]
              frame False {
                n141 = invoke class="App" method="Project.New"(error in=w409) -> (error out=w410:errorcluster, "Project:New"=w413:refnum<vi>)  [unwired: 2 in, 1 out]
                n142 = invoke class="Project" method="Open Window"(reference=w413, error in=w410) -> (reference out=w412:refnum<vi>, error out=w411:errorcluster)  [unwired: 1 in, 1 out]
              }
              frame True {
                n143 = Index Array(array=w416, index=w417) -> (element=w415:refnum<vi>)
              }
            }
            n144 = property class="Project"(reference=w403, error in=w400) -> (error out=w396:errorcluster, "My Computer"=w402:refnum<vi>, "App Ref"=w401:refnum<vi>)  [unwired: 1 out]
            n145 = Bundle By Name(cluster=w399, "My Computer Ref"=w402, "Application Ref"=w401) -> (w398:refnum<class "Springboard TLB`.lvclass">)
          }
        }
      }
      frame "Open Original Library" {
        n146 = case shown="\"Undo\"" w418 {
          tunnel: w422 -> [w425 w587]
          tunnel: [w425 w586] -> w421
          tunnel: w420 -> [w427 w585]
          tunnel: [w426 w584] -> w419
          frame "Undo" {
            n147 = Unbundle By Name(w425) -> ("Project Selection"=w424:u16)
            n148 = case shown="0" w424 {
              tunnel: w427 -> [w428 w434]
              tunnel: [w428 w430] -> w426
              tunnel: w425 -> [_ w429]
              frame Default {
              }
              frame 0 {
                # "close project that we tried to add the template to"
                n149 = property class="App"(error in=w434) -> (error out=w433:errorcluster, "Project"=w441:refnum<vi>[])  [unwired: 1 in, 1 out]
                n150 = for {
                  tunnel: w441 -> [w459] mode=indexing
                  tunnel: [w455] -> w440 mode=indexing if=w451
                  tunnel: [w453] -> w439 mode=indexing if=w451
                  tunnel: w433 -> [w450]
                  tunnel: [w447] -> w432
                  stop <- w447 stop-if-true
                  n151 = property class="Project"(reference=w459, error in=w450) -> (reference out=w453:refnum<vi>, error out=w449:errorcluster, "Name"=w458:string)
                  n152 = xnode "Match Regular Expression"("input string"=w458, "regular expression"="Untitled Project", "error in"=w449) -> ("after match"=w456:string, "offset past match"=w454:i32, "error out"=w448:errorcluster)  [unwired: 3 in, 2 out]
                  n153 = Less Than 0?(x=w454) -> (x < 0?=w452:bool)
                  n154 = Not(x=w452) -> (.not. x?=w451:bool)
                  n155 = case shown="True" w451 {
                    tunnel: w456 -> [_ w466]
                    tunnel: [_ w463] -> w455
                    tunnel: w448 -> [w460 w462]
                    tunnel: [w460 w461] -> w447
                    frame False {
                    }
                    frame True {
                      n156 = call <vilib>:"Trim Whitespace.vi"("string"=w466) -> ("trimmed string"=w465:string)  [unwired: 1 in]
                      n157 = Scan From String(input string=w465, error in=w462, default 1=u32 0) -> (error out=w461:errorcluster, output 1=w463:u32)  [unwired: 2 in, 2 out]
                    }
                  }
                }
                n158 = Array Max & Min(array=w440) -> (max index (indices)=w438:i32)  [unwired: 3 out]
                n159 = Index Array(array=w439, index=w438) -> (element=w437:refnum<vi>)
                n160 = Not A Number/Path/Refnum?(number/path/refnum=w437) -> (NaN/Path/Refnum?=w436:bool)
                n161 = case shown="False" w436 {
                  tunnel: w437 -> [w445 _]
                  tunnel: w432 -> [w444 w446]
                  tunnel: [w443 w446] -> w431
                  frame False {
                    n162 = invoke class="Project" method="Close"(reference=w445, error in=w444) -> (error out=w443:errorcluster)  [unwired: 1 in, 2 out]
                  }
                  frame True {
                  }
                }
                n163 = Unbundle By Name(w429) -> ("Library Path"=w442:refnum<vi>, "Library Path"=w435:path)
                n164 = property class="Path"(reference=w442, error in=w431, "Value"=w435) -> (error out=w430:errorcluster)  [unwired: 1 out]
              }
            }
          }
          frame Default {
            n165 = Unbundle By Name(w587) -> ("Library Path"=w590:path, "Application Ref"=w589:refnum<vi>)
            n166 = invoke class="App" method="Library.Open"(reference=w589, error in=w585, "path"=w590) -> (error out=w584:errorcluster, "Open Library"=w588:refnum<vi>)  [unwired: 1 in, 2 out]
            n167 = Bundle By Name(cluster=w587, "Reference Library Ref"=w588) -> (w586:refnum<class "Springboard TLB`.lvclass">)
          }
        }
      }
      frame "Save Copy Library" {
        n168 = case shown="Default" w591 {
          tunnel: w595 -> [w599 w633]
          tunnel: w594 -> [w605 w632]
          tunnel: [w605 w630] -> w593
          tunnel: [w600 w631] -> w592
          frame "Undo" {
            n169 = Unbundle By Name(w605) -> ("My Computer Ref"=w603:refnum<vi>, "Copied Library Path"=w597:path)
            n170 = Strip Path(path=w597) -> (name=w598:string)  [unwired: 1 out]
            n171 = invoke class="TargetItem" method="Get All Descendents"(reference=w603, error in=w599) -> (error out=w602:errorcluster, "All Descendents"=w604:refnum<vi>[])  [unwired: 5 in, 5 out]
            n172 = for {
              tunnel: w604 -> [w613] mode=indexing
              tunnel: w602 -> [w610]
              tunnel: [w608] -> w601 mode=indexing
              tunnel: w598 -> [w607]
              n173 = property class="ProjectItem"(reference=w613, error in=w610) -> (reference out=w611:refnum<vi>, error out=w609:errorcluster, "Name"=w606:string)
              n174 = Equal?(x=w606, y=w607) -> (x = y?=w612:bool)
              n175 = case shown="False" w612 {
                tunnel: w611 -> [_ w616]
                tunnel: w609 -> [w614 w615]
                tunnel: [w614 w617] -> w608
                frame False {
                }
                frame True {
                  n176 = invoke class="ProjectItem" method="Delete"(reference=w616, error in=w615) -> (error out=w617:errorcluster)  [unwired: 1 in, 2 out]
                }
              }
            }
            n177 = Merge Errors(w601) -> (w600:errorcluster)
          }
          frame Default {
            n178 = Unbundle By Name(w632) -> ("Reference Library Ref"=w634:refnum<vi>, "My Computer Ref"=w635:refnum<vi>)
            n179 = Unbundle By Name(w632) -> ("Destination Folder"=w629:path, "New TLB Name"=w618:string)
            n180 = call <vilib>:"Set Busy.vi"("error in (no error)"=w633) -> ("error out"=w623:errorcluster)  [unwired: 9 in, 1 out]
            n181 = invoke class="Library" method="Save a Copy"(reference=w634, error in=w623, "Path"=w629, "New Name"=w618) -> (reference out=w624:refnum<vi>, error out=w619:errorcluster, "New Lib Path"=w622:path)  [unwired: 2 in, 3 out]
            n182 = invoke class="TargetItem" method="AddFile"(reference=w635, error in=w619, "Path"=w622) -> (error out=w626:errorcluster, "AddFile"=w625:refnum<vi>)  [unwired: 1 in, 2 out]
            n183 = Close Reference(reference=w624, error in (no error)=w626) -> (error out=w620:errorcluster)
            n184 = Close Reference(reference=w625, error in (no error)=w620) -> (error out=w621:errorcluster)
            n185 = Unbundle By Name(w621) -> ("status"=w628:bool)
            n186 = call <vilib>:"Unset Busy.vi"("error in (no error)"=w621) -> ("error out"=w631:errorcluster)  [unwired: 10 in]
            n187 = Not(x=w628) -> (.not. x?=w627:bool)
            n188 = Bundle By Name(cluster=w632, "Build Complete"=w627, "Copied Library Path"=w622) -> (w630:refnum<class "Springboard TLB`.lvclass">)
          }
        }
      }
      frame "Open Copied Library" {
        n189 = case shown="Default" w636 {
          tunnel: w640 -> [w643 w652]
          tunnel: [w643 w648] -> w639
          tunnel: [w642 w647] -> w638
          tunnel: w637 -> [w642 w646]
          frame "Undo" {
          }
          frame Default {
            n190 = Unbundle By Name(w652) -> ("Copied Library Path"=w656:path, "Application Ref"=w655:refnum<vi>)
            n191 = call <vilib>:"Set Busy.vi"("error in (no error)"=w646) -> ("error out"=w657:errorcluster)  [unwired: 9 in, 1 out]
            n192 = invoke class="App" method="Library.Open"(reference=w655, error in=w657, "path"=w656) -> (error out=w653:errorcluster, "Open Library"=w654:refnum<vi>)  [unwired: 1 in, 2 out]
            n193 = property class="Library"(reference=w654, error in=w653) -> (error out=w645:errorcluster, "Children[]"=w650:refnum<vi>[])  [unwired: 1 out]
            n194 = call "Get Recursive Owned VIs List.vi"("Parent[]"=w650, "error in"=w645) -> ("Children[]"=w651:refnum<vi>[], "error out"=w644:errorcluster)  [unwired: 12 in]
            n195 = Build Array (concatenate)(w650, w651) -> (w649:refnum<vi>[])
            n196 = Bundle By Name(cluster=w652, "Copied Library Ref"=w654, "Owned Items[]"=w649) -> (w648:refnum<class "Springboard TLB`.lvclass">)
            n197 = flat-sequence {
              tunnel: [w658] -> w647
              tunnel: w644 -> [w658]
              frame #0 {
                n198 = call <vilib>:"Unset Busy.vi"() -> ()  [unwired: 11 in, 1 out]
              }
            }
          }
        }
      }
      frame "Rename TMPL VIs" {
        n199 = case shown="Default" w660 {
          tunnel: w663 -> [w666 w667]
          tunnel: w662 -> [w665 w670]
          tunnel: [w665 w668] -> w661
          tunnel: [w666 w667] -> w659
          frame "Undo" {
          }
          frame Default {
            n200 = Unbundle By Name(w667) -> ("Owned Items[]"=w673:refnum<vi>[], "New TLB Name"=w672:string)
            n201 = call "Find and Rename VIs.vi"("Owned Items[]"=w673, "new name"=w672, "name to replace"="TMPL") -> ("error out"=w671:errorcluster)  [unwired: 12 in]
            n202 = Merge Errors(w670, w671) -> (w668:errorcluster)
          }
        }
      }
      frame "Rename TMPL Libraries" {
        n203 = case shown="Default" w676 {
          tunnel: w678 -> [w681 w683]
          tunnel: w677 -> [w680 w686]
          tunnel: [w681 w683] -> w675
          tunnel: [w680 w682] -> w674
          frame "Undo" {
          }
          frame Default {
            n204 = Unbundle By Name(w683) -> ("Application Ref"=w687:refnum<vi>, "Owned Items[]"=w689:refnum<vi>[], "New TLB Name"=w688:string)
            n205 = call "Find and Rename Libraries.vi"("Owned Items[]"=w689, "Private Data.Application Ref"=w687, "new name"=w688, "name to replace"="TMPL") -> ("error out"=w685:errorcluster)  [unwired: 11 in]
            n206 = Merge Errors(w686, w685) -> (w682:errorcluster)
          }
        }
      }
      frame "/*********SHUTDOWN********/" {
      }
      frame "Exit" {
        w695 = refnum<class> refnum  # event data
        # "Don't wire 'Error In'\nMust Execute Regardless"
        n207 = Unbundle By Name(w699) -> ("Exit Event"=w693:refnum<user-event>)
        n208 = Generate User Event(user event=w693, event data cluster=w695) -> (error out=w698:errorcluster)  [unwired: 2 in, 1 out]
        n209 = Merge Errors(w696, w698) -> (w697:errorcluster)
      }
      frame "/*********ERRor Handler********/" {
      }
      frame "ERR::Log" {
        n210 = Unbundle By Name(w707) -> ("Error Handler"=w709:refnum<class "TLB` Error Handler.lvclass">)
        n211 = call-dynamic "Log.vi"("error handler in"=w709) -> ("error handler out"=w708:refnum<class "TLB` Error Handler.lvclass">, "error out"=w705:errorcluster)  [unwired: 13 in]
        n212 = Bundle By Name(cluster=w707, "Error Handler"=w708) -> (w706:refnum<class "Springboard TLB`.lvclass">)
        n213 = Merge Errors(w704, w705) -> (w703:errorcluster)
      }
      frame "ERR::Dialog" {
        n214 = Unbundle By Name(w718) -> ("Error Handler"=w714:refnum<class "TLB` Error Handler.lvclass">)
        n215 = call-dynamic "Dialog.vi"("error handler in"=w714, "trigger queue in"=w711) -> ("error handler out"=w713:refnum<class "TLB` Error Handler.lvclass">, "error out"=w712:errorcluster)  [unwired: 12 in]
        n216 = Merge Errors(w716, w712) -> (w715:errorcluster)
        n217 = Bundle By Name(cluster=w718, "Error Handler"=w713) -> (w717:refnum<class "Springboard TLB`.lvclass">)
      }
      frame Default {
        n218 = xnode "Error Ring"("parameter 0"=w720) -> ("error out"=w719:errorcluster)
      }
    }
    n219 = call "State Logic.vi"("TLB' data in"=w91, "process state logic enable"=w88, "trigger queue in"=w81, "action queue in"=w95, "error in"=w87) -> ("TLB' data out"=w92:refnum<class "Springboard TLB`.lvclass">, "error out"=w90:errorcluster)  [unwired: 9 in]
  }
  n220 = while {
    tunnel: w9 -> [w734]
    tunnel: [w730] -> w7
    i -> [w733]
    stop <- w732 stop-if-true
    # "UI Display Handler Loop"
    n221 = event shown="[0] Timeout" {
      selector: w734 -> [_ _ _ _ _]
      dyn-events: [_ _ _ _ _] -> w730
      timeout: 100 -> [_ _ _ _ _]
      tunnel: w733 -> [_ _ _ _ _]
      tunnel: [_ _ _ TRUE _] -> w732
      event Timeout {
        n222 = event-data() -> ()  [unwired: 2 out]
      }
      event User Event {
        n223 = event-data() -> ("State"=→"State":string)  [unwired: 1 out]
      }
      event User Event {
        n224 = event-data() -> ("Status"=→"Status":string)  [unwired: 1 out]
      }
      event User Event {
        n225 = event-data() -> ()  [unwired: 2 out]
      }
      event User Event {
        n226 = event-data() -> ("Application Name"=→"Application Name":string)  [unwired: 1 out]
      }
    }
  }
  n227 = while {
    tunnel: w11 -> [w742]
    tunnel: [w741] -> w14
    tunnel: w6 -> [w739]
    i -> [w740]
    stop <- w743 stop-if-true
    # "Event Handler Loop"
    n228 = event shown="[5] \"Build\": Value Change" {
      selector: w742 -> [_ _ _ _ _ _]
      dyn-events: [_ _ _ _ _ _] -> w741
      timeout: _ -> [_ _ _ _ _ _]
      tunnel: [_ _ _ TRUE ("NewVal") _ _] -> w743
      tunnel: w740 -> [_ _ _ _ _ _]
      tunnel: w739 -> [w744 w747 _ w758 w762 w765]
      event Panel Close? {
        w746 = TRUE  # Discard?
        n229 = event-data() -> ()  [unwired: 2 out]
        n230 = call "EnQueue Trigger.vi"("trigger queue in"=w744, "system trigger"=System_Trigger."<Close Application>" ("System Trigger")) -> ()  [unwired: 12 in, 2 out]
        n231 = event-data("Discard?"=w746) -> ()  [unwired: 1 in, 1 out]
      }
      event "Cancel": Value Change {
        n232 = event-data() -> ()  [unwired: 7 out]
        n233 = call "EnQueue Trigger.vi"("trigger queue in"=w747, "system trigger"=System_Trigger."<Close Application>" ("System Trigger")) -> ()  [unwired: 12 in, 2 out]
      }
      event Mouse Down {
        n234 = event-data() -> ("Button"=w749:u16, "Mods.Double Click"=w750:bool)  [unwired: 1 out]
        n235 = Equal?(x=u16 2, y=w749) -> (x = y?=w752:bool)
        n236 = Compound Arithmetic op=AND(w752, w750) -> (w751:bool)
        n237 = case "Toggle Menu Visibility :: double RIGHT click on logo" shown="True" w751 {
          frame False {
          }
          frame True {
            n238 = property class="VI"() -> (reference out=w756:refnum<vi>, "TB.Visible"=w755:bool)  [unwired: 2 in, 1 out]
            n239 = Not(x=w755) -> (.not. x?=w754:bool)
            n240 = property class="VI"(reference=w756, "TB.Visible"=w754, "Front Panel.ShowMenuBar"=w754) -> ()  [unwired: 1 in, 2 out]
          }
        }
      }
      event User Event {
        n241 = event-data() -> ()  [unwired: 2 out]
        n242 = call "EnQueue Trigger.vi"("trigger queue in"=w758, "system trigger"=System_Trigger."<Close Application>" ("System Trigger")) -> ()  [unwired: 12 in, 2 out]
      }
      event Value Change {
        n243 = event-data() -> ()  [unwired: 2 out]
        n244 = call "EnQueue Trigger.vi"("trigger queue in"=w762, "system trigger"=System_Trigger."<Cache User Parameters>" ("System Trigger")) -> ("trigger queue out"=w761:refnum<queue>)  [unwired: 12 in, 1 out]
        n245 = event "use this event case to register a SPEICIFIC 'User Parameter' for a SPECIFIC action" shown="[0] Timeout" {
          selector: _ -> [_]
          dyn-events: _ -> [_]
          timeout: 0 -> [_]
          tunnel: w761 -> [_]
          event Timeout {
            n246 = event-data() -> ()  [unwired: 1 in, 1 out]
          }
        }
      }
      event "Build": Value Change {
        n247 = event-data() -> ()  [unwired: 2 out]
        n248 = call "EnQueue Trigger.vi"("trigger queue in"=w765, "system trigger"=System_Trigger."Create New") -> ()  [unwired: 12 in, 2 out]
      }
    }
  }
  n249 = while {
    shift-right: [w775] -> _
    shift-left: T2."Close Display" -> [w768]
    tunnel: w14 -> [w773]
    tunnel: w8 -> [w774]
    tunnel: [w771] -> w16
    shift-right: [w770] -> w4
    shift-left: w13 -> [w772]
    tunnel: w7 -> [w769]
    i -> [w766]
    stop <- w767 stop-if-true
    # "Application Close"
    n250 = case shown="\"Close Display\"" w768 {
      tunnel: [w781 w787 w792] -> w771
      tunnel: [w780 w786 w789] -> w770
      tunnel: [w782 _ w791] -> _
      tunnel: w774 -> [w781 w787 w792]
      tunnel: w773 -> [w782 w785 w791]
      tunnel: w772 -> [w780 w786 w789]
      tunnel: w769 -> [w779 w783 w790]
      tunnel: [w779 _ w790] -> _
      frame "Close Display" {
        n251 = Unbundle By Name(w780) -> ("MAIN VI Refnum"=w776:refnum<vi>)
        n252 = invoke class="VI" method="FP.Open"(reference=w776, "Activate"=TRUE ("Activate?"), "State"=T10."Hidden") -> ()  [unwired: 2 in, 5 out]
      }
      frame "Clear References" {
        n253 = Unregister For Events(event registration refnum=w783) -> ()  [unwired: 1 in, 1 out]
        n254 = Unbundle By Name(w786) -> ("Framework Events"=w784:T5)
        n255 = Unregister For Events(event registration refnum=w785) -> ()  [unwired: 1 in, 1 out]
        n256 = call "Destroy CORE UI Display Events.vi"("UI display events in"=w784) -> ()  [unwired: 14 in, 1 out]
      }
      frame "Close Error Handler" {
        n257 = Unbundle By Name(w789) -> ("Error Handler"=w788:refnum<class "TLB` Error Handler.lvclass">)
        n258 = call-dynamic "Close.vi"("error handler in"=w788) -> ()  [unwired: 14 in, 1 out]
      }
    }
    n259 = call "Enum Loop Complete.vi"("Current State Enum"=w768, "Itteration"=w766) -> ("Loop Complete?"=w767:bool)  [unwired: 12 in, 1 out]
    n260 = Increment(x=w768) -> (x+1=w775:T2)
  }
  n261 = Unbundle By Name(w4) -> ("Terminate Error"=w3:errorcluster)
  n262 = disable-structure shown="RUN_TIME_ENGINE==True" {
    disable-tunnel: [w793 w794] -> w2
    disable-tunnel: w16 -> [w793 w795]
    frame condition #0 (active) {
    }
    frame condition #1 {
      n263 = flat-sequence {
        tunnel: [w796] -> w794
        tunnel: w795 -> [w796]
        frame #0 {
          n264 = Quit LabVIEW() -> ()  [unwired: 1 in]
        }
      }
    }
  }
  n265 = Merge Errors(w3, w2) -> (→"error out":errorcluster)
